vi "Resolve Selected Paths.vi"(9 "File Items":T1(array[cluster]), 11 "Selected Tags":string[](array[string])) -> (3 "Files to Push":string[](array[string]))   [LabVIEW 2025]
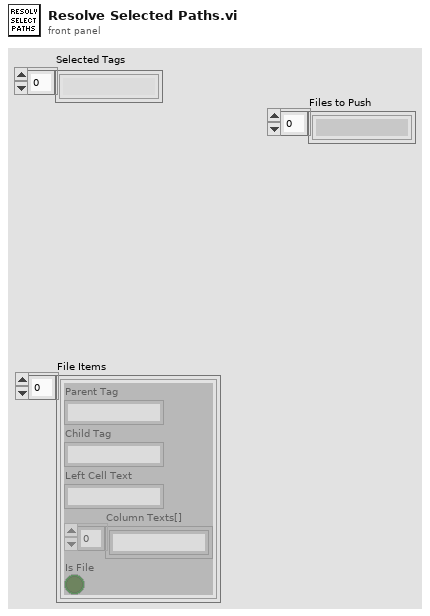
[diagram p1: front panel]
types:
  T1 = cluster{"Parent Tag":string, "Child Tag":string, "Left Cell Text":string, "Column Texts[]":string[], "Is File":bool}[]
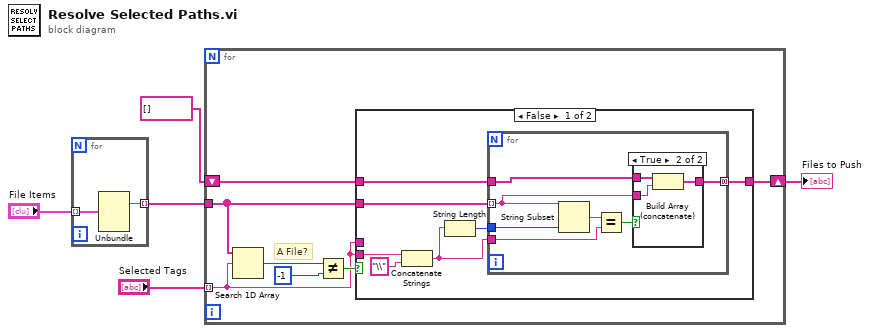
[diagram p0: block diagram]
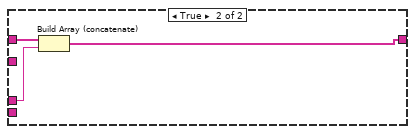
[diagram p3: hidden frame]
diagram:
  n1 = for {
    tunnel: "File Items" -> [w7] mode=indexing
    tunnel: [w6] -> w1 mode=indexing
    n2 = Unbundle(w7) -> ("Child Tag"=w6:string)  [unwired: 4 out]
  }
  n3 = for {
    tunnel: "Selected Tags" -> [w8] mode=indexing
    tunnel: w1 -> [w9]
    shift-right: [w10] -> w3
    shift-left: string[] [] ("Selected Tags") -> [w11]
    # "A File?"
    n4 = Search 1D Array(1D array=w9, element=w8) -> (index of element=w14:i32)  [unwired: 1 in]
    n5 = Not Equal?(x=w14, y=-1) -> (x != y?=w12:bool)
    n6 = case shown="False" w12 {
      tunnel: w11 -> [w17 w35]
      tunnel: w8 -> [_ w34]
      tunnel: [w15 w33] -> w10
      tunnel: w8 -> [w21 _]
      tunnel: w9 -> [w19 _]
      frame False {
        n7 = Concatenate Strings(w21, "\\" ("string")) -> (w16:string)
        n8 = String Length(string=w16) -> (length=w18:i32)
        n9 = for {
          tunnel: w19 -> [w23] mode=indexing
          tunnel: w18 -> [w28]
          tunnel: w17 -> [w27]
          tunnel: w16 -> [w25]
          tunnel: [w22] -> w15 mode=concatenating
          n10 = String Subset(string=w23, length (rest)=w28) -> (substring=w26:string)  [unwired: 1 in]
          n11 = Equal?(x=w26, y=w25) -> (x = y?=w24:bool)
          n12 = case shown="True" w24 {
            tunnel: w27 -> [w29 w32]
            tunnel: w23 -> [_ w31]
            tunnel: [w29 w30] -> w22
            frame False {
            }
            frame True {
              n13 = Build Array (concatenate)(w32, w31) -> (w30:string[])
            }
          }
        }
      }
      frame True {
        n14 = Build Array (concatenate)(w35, w34) -> (w33:string[])
      }
    }
  }
  "Files to Push" <- w3
